vi "TSP-搜索树形列表.vi"(8 "error in (no error)":errorcluster caption="错误输入（无错误）", 10 "NG/OK":string(combo)="Image", 11 "检索条件":string(combo)="CCD6") -> (0 "错误输出":errorcluster, 2 "项缩进层次":i32[](array[numeric]), 3 "项名称":string[](array[string]), 4 "All Files in Dir":path[](array[path]) caption="目录中的所有文件", 5 "文件夹名":string[](array[string]))   [LabVIEW 2017]
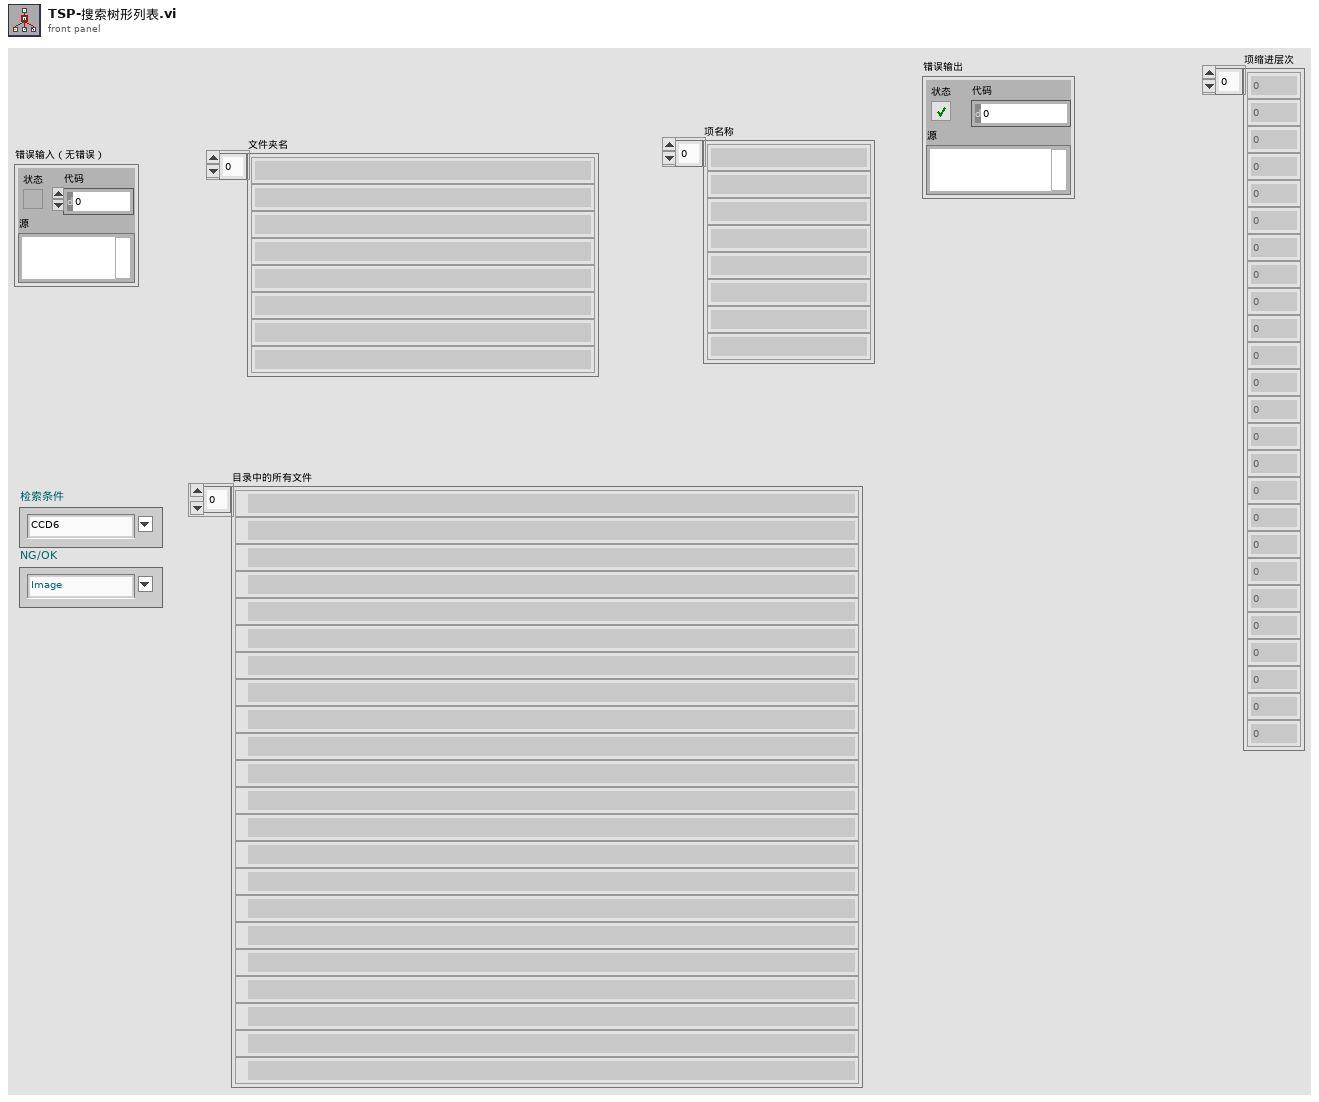
[diagram p1: front panel]
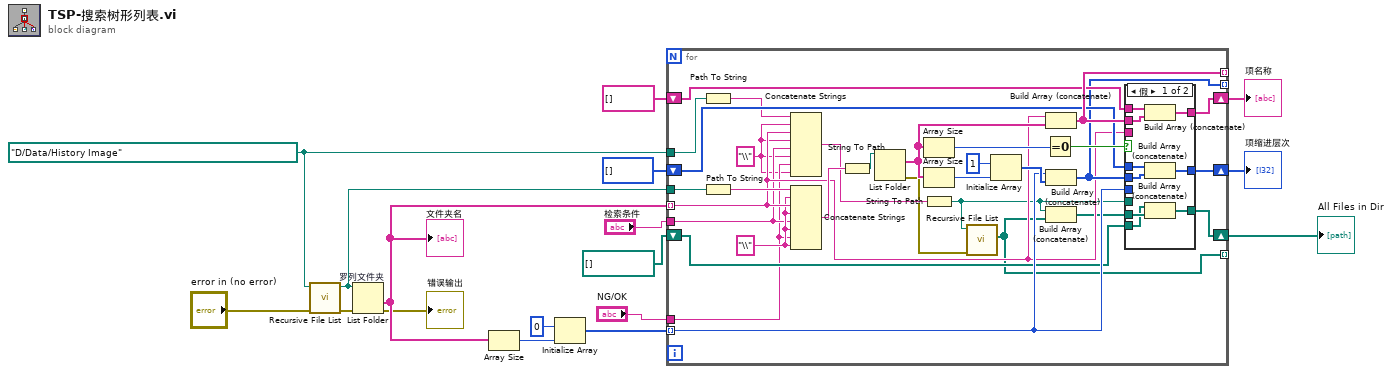
[diagram p0: block diagram]
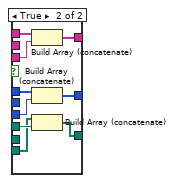
[diagram p2: hidden frame]
diagram:
  w2 = path "D:/Data/History Image" ("Folder Path")
  n1 = call <vilib>:"Recursive File List.vi"("error in (no error)"="error in (no error)", "Folder Path"=w2) -> ("error out"=w17:errorcluster, "dup Folder Path"=w1:path)  [unwired: 5 in, 3 out]
  n2 = List Folder "罗列文件夹"(path=w1, error in=w17) -> (folder names=w16:string[], error out=→"错误输出":errorcluster)  [unwired: 2 in, 2 out]
  "文件夹名" <- w16
  n3 = Array Size(array=w16) -> (size(s)=w13:i32)
  n4 = Initialize Array(0 ("维数大小"), w13) -> (w15:i32[])
  n5 = for {
    tunnel: w16 -> [w27] mode=indexing
    tunnel: w1 -> [w48]
    tunnel: [w37] -> _ mode=indexing
    tunnel: w15 -> [w32] mode=indexing
    tunnel: [w33] -> _ mode=indexing
    shift-right: [w38] -> w11
    shift-left: string[] [] -> [w36]
    shift-right: [w34] -> w9
    shift-left: i32[] [] -> [w35]
    shift-right: [w30] -> w5
    shift-left: path[] [] -> [w31]
    tunnel: w2 -> [w29]
    tunnel: [w25] -> _ mode=indexing
    tunnel: "检索条件" -> [w21]
    tunnel: "NG/OK" -> [w20]
    w19 = "\\" ("字符串")
    w22 = "\\" ("字符串")
    n6 = Path To String(path=w29) -> (string=w28:string)
    n7 = Path To String(path=w48) -> (string=w47:string)
    n8 = Concatenate Strings(w28, w19, w27, w19, w21, w19, w20, w19) -> (w26:string)
    n9 = Concatenate Strings(w47, w22, w27, w22, w21, w22, w20, w22) -> (w46:string)
    n10 = String To Path(string=w46) -> (path=w45:path)
    n11 = List Folder(path=w45) -> (filenames=w40:string[], error out=w18:errorcluster)  [unwired: 3 in, 2 out]
    n12 = Array Size(array=w40) -> (size(s)=w41:i32)
    n13 = Array Size(array=w40) -> (size(s)=w42:i32)
    n14 = String To Path(string=w26) -> (path=w24:path)
    n15 = call <vilib>:"Recursive File List.vi"("error in (no error)"=w18, "Folder Path"=w24) -> ("All Files in Dir"=w25:path[])  [unwired: 5 in, 4 out]
    n16 = Initialize Array(1 ("维数大小"), w42) -> (w44:i32[])
    n17 = Equal To 0?(x=w41) -> (x = 0?=w39:bool)
    n18 = Build Array (concatenate)(w27, w40) -> (w37:string[])
    n19 = Build Array (concatenate)(w32, w44) -> (w33:i32[])
    n20 = Build Array (concatenate)(w24, w25) -> (w23:path[])
    n21 = case shown="假" w39 {
      tunnel: w36 -> [w57 w65]
      tunnel: [w55 w64] -> w38
      tunnel: w37 -> [w56 _]
      tunnel: w35 -> [w53 w62]
      tunnel: [w52 w61] -> w34
      tunnel: w33 -> [w54 _]
      tunnel: w27 -> [_ w66]
      tunnel: w32 -> [_ w63]
      tunnel: w31 -> [w50 w59]
      tunnel: [w49 w58] -> w30
      tunnel: w24 -> [_ w60]
      tunnel: w23 -> [w51 _]
      frame False {
        n22 = Build Array (concatenate)(w57, w56) -> (w55:string[])
        n23 = Build Array (concatenate)(w53, w54) -> (w52:i32[])
        n24 = Build Array (concatenate)(w50, w51) -> (w49:path[])
      }
      frame True {
        n25 = Build Array (concatenate)(w65, w66) -> (w64:string[])
        n26 = Build Array (concatenate)(w62, w63) -> (w61:i32[])
        n27 = Build Array (concatenate)(w59, w60) -> (w58:path[])
      }
    }
  }
  "项名称" <- w11
  "项缩进层次" <- w9
  "All Files in Dir" <- w5
